vi "FTW-JSON-Interpret-Boolean.vi"(1 "JSON Boolean":string) -> (0 "LabVIEW Boolean":bool)   [LabVIEW 2015]
panel:
  # "Inputs"
  # "Outputs"
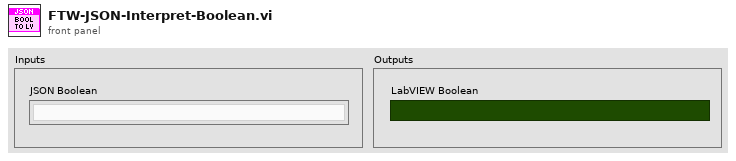
[diagram p1: front panel]
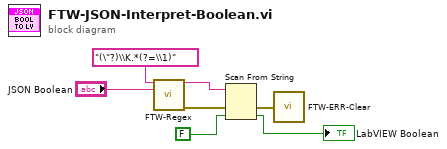
[diagram p0: block diagram]
diagram:
  n1 = call "FTW-Regex.vi"("Regular Expression"="(\"?)\\K.*(?=\\1)", "Input String"="JSON Boolean") -> ("Match"=w3:string, "error out"=w2:errorcluster)  [unwired: 9 in, 3 out]
  n2 = Scan From String(input string=w3, error in=w2, default 1=FALSE ("Affirmative?")) -> (error out=w6:errorcluster, output 1=→"LabVIEW Boolean":bool)  [unwired: 2 in, 2 out]
  n3 = call "FTW-ERR-Clear.vi"("error to snuff"=w6) -> ()  [unwired: 1 out]
